vi "图像像素操作.vi"() -> ()   [LabVIEW 2018]
uses:
  <vilib>/vision/NI_Vision_Development_Module.lvlib
panel:
  out "Pixels Line (I16)":i16[](array[numeric])
  out "Image":T1(plugin-control)
  out "error out":errorcluster
  out "Pixels (U8)":u8[](array[numeric])
  out "Pixel Value (U8)":u8
  in  "路径":path
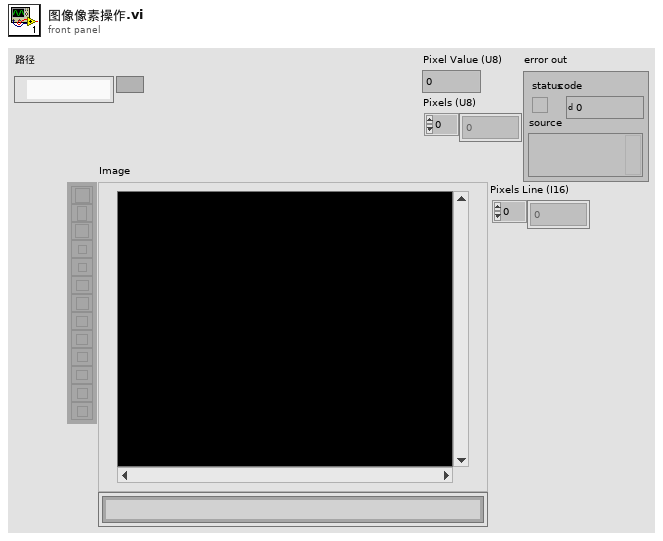
[diagram p1: front panel]
types:
  T1 = typedef "IMAQ Image.ctl" = refnum<image>
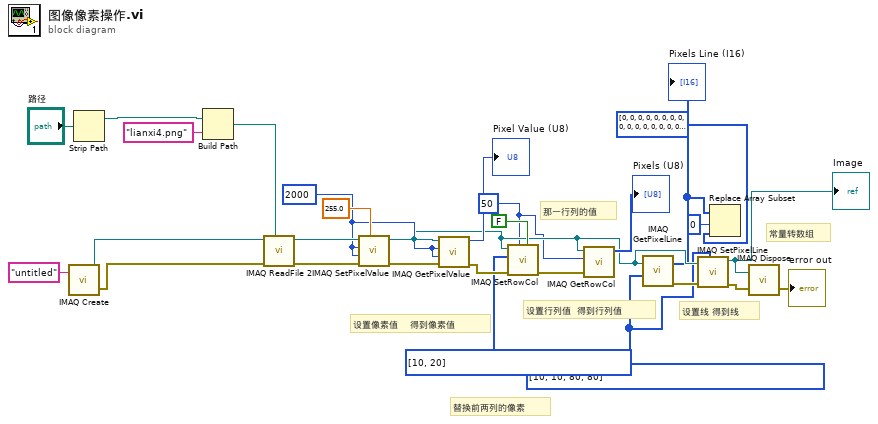
[diagram p0: block diagram]
diagram:
  w3 = i32[] [10, 10, 80, 80] ("Line Coordinates")
  w2 = 50 ("Number")
  w17 = 2000 ("X Coordinate")
  # "常量转数组"
  # "设置线 得到线"
  # "替换前两列的像素"
  # "那一行列的值"
  # "设置行列值  得到行列值"
  # "设置像素值    得到像素值"
  n1 = call "IMAQ Create"("Image Name"="untitled") -> ("New Image"=w23:T1, "error out"=w24:errorcluster)  [unwired: 4 in]
  n2 = Strip Path(path="路径") -> (stripped path=w26:path)  [unwired: 1 out]
  n3 = Build Path(base path=w26, name or relative path="lianxi4.png" ("名称或相对路径")) -> (appended path=w22:path)
  n4 = call "IMAQ ReadFile 2"("File Path"=w22, "error in (no error)"=w24, "Image"=w23) -> ("error out"=w20:errorcluster, "Image Out"=w21:T1)  [unwired: 4 in, 3 out]
  n5 = call "IMAQ SetPixelValue"("Pixel Value"=sgl 255.0, "error in (no error)"=w20, "Y Coordinate"=w17, "X Coordinate"=w17, "Image"=w21) -> ("error out"=w18:errorcluster, "Image Out"=w6:T1)  [unwired: 5 in]
  n6 = call "IMAQ GetPixelValue"("Image"=w6, "X Coordinate"=w17, "Y Coordinate"=w17, "error in (no error)"=w18) -> ("Pixel Value (U8)"=→"Pixel Value (U8)":u8, "error out"=w14:errorcluster)  [unwired: 2 in, 3 out]
  n7 = call "IMAQ SetRowCol"("Row / Column (Row)"=FALSE, "Number"=w2, "error in (no error)"=w14, "Pixels (U8)"=u8[] [10, 20], "Image"=w6) -> ("error out"=w12:errorcluster)  [unwired: 5 in, 1 out]
  n8 = call "IMAQ GetRowCol"("Image"=w6, "Number"=w2, "error in (no error)"=w12) -> ("Pixels (U8)"=→"Pixels (U8)":u8[])  [unwired: 3 in, 4 out]
  n9 = call "IMAQ GetPixelLine"("Line Coordinates"=w3, "Image"=w6) -> ("error out"=w5:errorcluster, "Pixels Line (I16)"=w1:i16[])  [unwired: 2 in, 3 out]
  "Pixels Line (I16)" <- w1
  n10 = call "IMAQ SetPixelLine"("Line Coordinates"=w3, "error in (no error)"=w5, "Image"=w6) -> ("error out"=w10:errorcluster, "Image Out"=w4:T1)  [unwired: 7 in]
  "Image" <- w4
  n11 = Replace Array Subset(array=w1, new element=u8[] [0, 0, 0, 0, 0, 0, 0, 0, 0, 0, 0, 0, 0, 0, 0, 0, 0, 0, 0, 0, 0, 0, 0, 0, 0, 0, 0, 0, 0, 0, 0, 0, 0, 0, 0, 0, 0, 0, 0, 0, 0, 0, 0, 0, 0, 0, 0, 0, 0, 0, 0, 0, 0, 0, 0, 0, 0, 0, 0, 0, 0, 0, 0, 0, 0, 0, 0, 0, 0, 0, 0, 0, 0, 0, 0, 0, 0, 0, 0, 0, 0, 0, 0, 0, 0, 0, 0, 0, 0, 0, 0, 0, 0, 0, 0, 0, 0, 0, 0, 0, 0] ("新元素/子数组"), index=0 ("索引")) -> ()  [unwired: 1 out]
  n12 = call "IMAQ Dispose"("Image"=w4, "error in (no error)"=w10) -> ("error out"=→"error out":errorcluster)  [unwired: 4 in]
